vi "Protocol.Main.vi"(10 "Parameters":variant, 11 "Process":refnum<class "Process.lvclass">) -> ()   [LabVIEW 2015, in "J1939 Addon Engine.lvlib"]
uses:
  J1939 Addon Engine.lvlib
  <vilib>/NI/NIVS Inline Async API/_VS Inline Async API/Process/Process.lvclass
  Types/Protocol.App Settings.ctl
  Shared/Types/XNET Settings.ctl
  Shared/Types/Monitor Settings.ctl
  Types/Protocol.XNET Refs.ctl
  <vilib>/NI Veristand/Custom Device API/Block Data Reference.ctl
  <vilib>/NI Veristand/Custom Device API/Data Reference.ctl
  Types/Main.Outgoing.Frame.Settings.ctl
  Shared/Types/Outgoing Event Trigger Types.ctl
  Types/Engine.DTC Settings.ctl
  Shared/Types/Compiled Simulated Settings.ctl
  Types/Engine.DTC FIFOs.ctl
  <vilib>/NI/NIVS Addon Network Comm/Engine/VeriStand Comm.lvclass/VeriStand Comm.ctl
  <vilib>/NI/NIVS Inline Async API/_VS Inline Async API/Process/Process.lvclass/Process.ctl
  Protocol.Read Queued Processed Outgoing Messages.vi
  Protocol.Convert Frame to NI-XNET CAN Frame.vi
  <vilib>/NI/NIVS Inline Async API/_VS Inline Async API/Process/Methods/Async.Processes.Report.vi
  Protocol.Process Incoming Messages.vi
  <vilib>/NI/NIVS Addon Network Comm/Engine/_SubVIs/Comm Connection Engine.vi
  <vilib>/NI/NIVS Addon Network Comm/Engine/_SubVIs/Comm Command Engine.vi
  Protocol.Process J1939 Incoming Messages.vi
  Protocol.RQST Lookup Table Act.vi
  <vilib>/NI/NIVS Addon Network Comm/Engine/Comm API/Read Command.vi
  Protocol.RQST Wait on Response.vi
  Protocol.RQST Wait on Multiple Requests.vi
  Shared/J1939 Utilities/Common Conversions.vi
  Shared/J1939 Utilities/SubVIs/Convert CAN Arb ID to J1939 ID.vi
  Protocol.Address Lookup Table Action.vi
  <vilib>/NI/NIVS Addon Network Comm/Engine/Comm API/Respond to Command.vi
  <vilib>/NI/NIVS Inline Async API/_VS Inline Async API/Error Handling Process/SubVIs/Error.ConvertArray.vi
  Protocol.Filter by Device Address.vi
  Protocol.Process Incoming Messages by PDU F.vi
  <vilib>/NI/STM/Connection Manager/TCP/Advanced/TCP Connection Manager (By Reference).vi
  <vilib>/Utility/error.llb/Clear Errors.vi
  <vilib>/NI/STM/Get Connection Reference.vi
  <vilib>/NI/STM/TCP/Get Connection Reference (TCP).vi
  <vilib>/NI/STM/Read Meta Data.vi
  <vilib>/NI/STM/TCP/Read Meta Data (TCP Ref).vi
  <vilib>/NI/AMC/Send Local Message.vi
  <vilib>/NI/Tools/Keyed Array/Add.vi
  <vilib>/NI/AMC/Read Next Message.vi
  <vilib>/NI/STM/Connection Manager/TCP/Advanced/TCP Check Connection (By Reference).vi
  Protocol.J1939 Filter by Device Address.vi
  <vilib>/NI/Tools/Keyed Array/Index.vi
  Shared/J1939 Utilities/Common Messages.vi
  Shared/J1939 Utilities/SubVIs/Request.vi
  Protocol.Parse Message Type.vi
  Protocol.RQST Look for Response.vi
  Shared/J1939 Utilities/SubVIs/Convert J1939 ID to CAN Arb ID.vi
  Shared/J1939 Utilities/SubVIs/Convert CAN Data (U32) to U8.vi
  Protocol.Get Simulated Previously Active DTCs.vi
  Protocol.Get Simulated Active DTCs.vi
  Shared/J1939 Utilities/SubVIs/Acknowledgement.vi
  Protocol.Send Reset Previously Active DTC to Main.vi
  Protocol.Send Reset Active DTC to Main.vi
  Protocol.Convert Signals to Frame by ID.vi
  <vilib>/NI/STM/SubVIs/Generate STM Error.vi
  <vilib>/NI/AMC/Create Single Message.vi
  <vilib>/NI/AMC/Update Message Routing Info.vi
  <vilib>/NI/Tools/Keyed Array/Map String.vi
  <vilib>/NI/AMC/Read Termination Message.vi
  Protocol.Convert Data to DTC Frame.vi
  <vilib>/NI/Tools/String/Get Case Matching.vi
  <vilib>/NI Veristand/Custom Device Tools/Custom Device Utility Library/NI VeriStand - Print Debug String.vi
  <vilib>/xnet/xnet.llb/XNET Clear.vi
  <vilib>/NI/NIVS Addon Network Comm/Engine/Process/Close Comm Refs.vi
  Protocol.Close References.vi
  <vilib>/xnet/xnet.llb/XNET Write.vi
  <vilib>/xnet/xnet.llb/XNET Write (Frame CAN).vi
  Protocol.Address Lookup Table.vi
  <vilib>/xnet/xnet.llb/XNET Convert.vi
  <vilib>/xnet/xnet.llb/XNET Convert (Signal to Frame CAN).vi
  <vilib>/xnet/xnet.llb/XNET Create Session.vi
  <vilib>/xnet/xnet.llb/XNET Create Session (Conversion).vi
  Protocol.RQST Lookup Table.vi
  <vilib>/xnet/xnet.llb/XNET Read.vi
  <vilib>/xnet/xnet.llb/XNET Read (Frame CAN).vi
  <vilib>/NI/STM/TCP/Read Meta Data (TCP Clst).vi
  <vilib>/NI/AMC/Destroy Message Queue.vi
  <vilib>/NI/STM/Write Message.vi
  <vilib>/NI/STM/TCP/Write Message (TCP).vi
  <vilib>/NI/AMC/Globals.vi
  <vilib>/NI/AMC/Send Message.vi
  <vilib>/NI/AMC/Create Message Queue.vi
  <vilib>/NI/NIVS Addon Network Comm/Shared/Comm Constants.vi
  <vilib>/NI/STM/Read Message.vi
  <vilib>/NI/STM/TCP/Read Message (TCP).vi
  <vilib>/xnet/xnet.llb/XNET Read (State CAN Comm).vi
  <vilib>/Utility/error.llb/Error Cluster From Error Code.vi
  <vilib>/NI/NIVS Addon Network Comm/Engine/VeriStand Comm.lvclass
  Shared/J1939 Addon Shared.lvlib
  <vilib>/NI VeriStand/Custom Device API/Custom Device API.lvlib
panel:
  out "error out":errorcluster
  # "CONTROL & MONITORING"
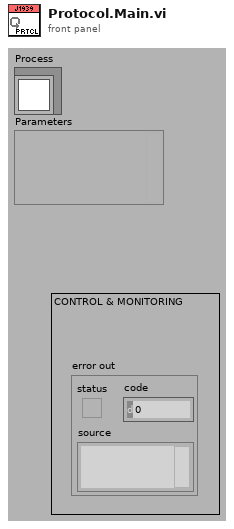
[diagram p1: front panel]
types:
  T1 = typedef "J1939 Addon Engine.lvlib/Protocol.App Settings.ctl" = cluster{"Name":string, "XNET.Settings":T2, "Monitor.Network":T3, "Data":T4[], "DTCs":T9[], "Sim.Nodes.LUT":variant, "Data.LUT":variant}
  T2 = typedef "J1939 Addon Shared.lvlib/XNET Settings.ctl" = cluster{"Database":refnum<k21>, "Cluster":refnum<k21>, "Port":string, "Baud rate [Bd]":u32, "Termination":u32, "Incoming Decimation":u32, "Outgoing Decimation":u32}
  T3 = typedef "J1939 Addon Shared.lvlib/Monitor Settings.ctl" = cluster{"Address":u8, "Name":u64, "Include DA":bool}
  T4 = typedef "J1939 Addon Engine.lvlib/Protocol.XNET Refs.ctl" = cluster{"Network":T3, "Incoming.Use":bool, "Incoming.Session":refnum<k21>, "Incoming.Refs":T5[], "Incoming.Values":dbl[], "Outgoing.Frames":T7[], "Outgoing.Initialize":bool, "Outgoing.Refs":T5[], "Outgoing.Values":dbl[], "Request.Table":refnum<k33>, "Timing.Use":bool, "Timing.Index":i32[], "Timing.Refs":T5[], "Timing.Values":dbl[], "Disable.Refs":T5[], "Disable.Values":dbl[], "Trigger.Refs":T5[], "Trigger.Values":dbl[]}
  T5 = typedef "Custom Device API.lvlib/Block Data Reference.ctl" = cluster{"Data Reference":T6, "Offset":u64, "Length":u64}
  T6 = typedef "Custom Device API.lvlib/Data Reference.ctl" = i32
  T7 = typedef "J1939 Addon Engine.lvlib/Main.Outgoing.Frame.Settings.ctl" = cluster{"Offset":u32, "Length":u32, "Cyclic":bool, "Disable.Index":i32, "Disable":bool, "Trigger":T8, "Trigger.Index":i32, "Session":refnum<k21>}
  T8 = typedef "J1939 Addon Shared.lvlib/Outgoing Event Trigger Types.ctl" = enum16{"Channel value change", "Trigger channel (not zero)", "Channel value change or trigger channel (not zero)", "Trigger channel (any value change)", "Channel value change or trigger channel (any value change)"}
  T9 = typedef "J1939 Addon Engine.lvlib/Engine.DTC Settings.ctl" = cluster{"Data":T10, "FIFOs":T11}
  T10 = typedef "J1939 Addon Shared.lvlib/Compiled Simulated Settings.ctl" = cluster{"DM1.Ref":T5[], "DM1.Value":dbl[], "DM1.Enable.Ref":T5[], "DM1.Enable.Value":dbl[], "DM2.Ref":T5[], "DM2.Value":dbl[], "DM2.Enable.Ref":T5[], "DM2.Enable.Value":dbl[]}
  T11 = typedef "J1939 Addon Engine.lvlib/Engine.DTC FIFOs.ctl" = cluster{"DM1.Data":refnum<k33>, "DM1.Enable":refnum<k33>, "DM2.Data":refnum<k33>, "DM2.Enable":refnum<k33>, "DM1.Reset":refnum<k33>, "DM2.Reset":refnum<k33>}
  T12 = typedef "J1939 Addon Engine.lvlib/Protocol.Configuration.ctl" = cluster{"Refs":T13, "XNET":T16, "Comm":refnum<class "VeriStand Comm.lvclass">, "Process":refnum<class "Process.lvclass">, "Name":string, "InternalCmd":T17, "InternalResp":T18, "Resp.Data":dbl[]}
  T13 = typedef "J1939 Addon Engine.lvlib/Protocol.Refs.ctl" = cluster{"Processed Outgoing":refnum<queue>, "Simulated Addresses LUT":variant, "Data LUT":variant, "RequestDataTables":refnum<k33>[], "RQST":T14, "Address LUT":T15, "Addresses":u8[], "Monitor Address":u8}
  T14 = typedef "J1939 Addon Engine.lvlib/Protocol.RQST Lookup Table Reference.ctl" = refnum<data-value>
  T15 = typedef "J1939 Addon Engine.lvlib/Protocol.Address Table Reference.ctl" = refnum<data-value>
  T16 = typedef "J1939 Addon Engine.lvlib/Protocol.XNET Settings.ctl" = cluster{"Raw CAN In":refnum<k21>, "Raw Frames out":refnum<k21>[], "Raw J1939 In":refnum<k21>}
  T17 = typedef "Data Access Engine.lvlib/Data Access Engine.lvclass/Read.DVR.ctl" = refnum<data-value>
  T18 = typedef "Data Access Engine.lvlib/Data Access Engine.lvclass/Write.DVR.ctl" = refnum<data-value>
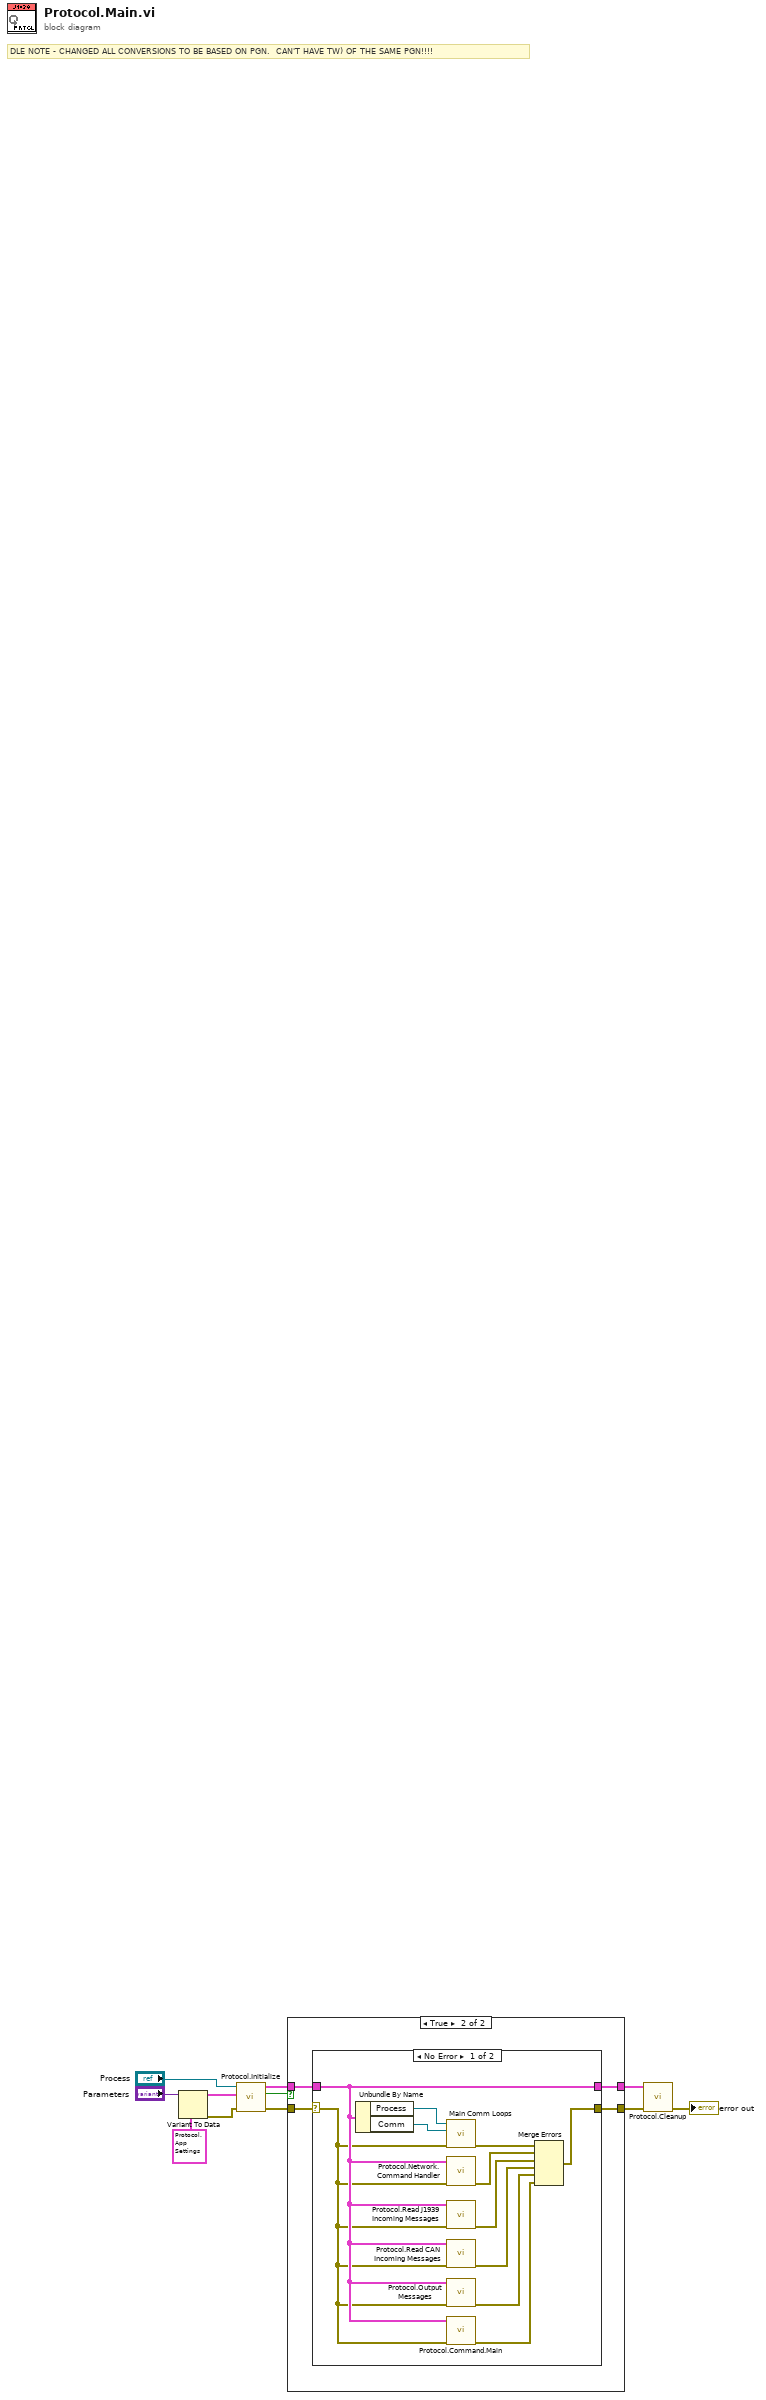
[diagram p0: block diagram]
diagram:
  # "DLE NOTE - CHANGED ALL CONVERSIONS TO BE BASED ON PGN.  CAN'T HAVE TW) OF THE SAME PGN!!!!"
  n1 = Variant To Data(type=T1 {"Name"="", "XNET.Settings"={"Database"="", "Cluster"="", "Port"="", "Baud rate [Bd]"=0, "Termination"=0, "Incoming Decimation"=0, "Outgoing Decimation"=1}, "Monitor.Network"={"Address"=0, "Name"=0, "Include DA"=FALSE}, "Data"=[], "DTCs"=[], "Sim.Nodes.LUT"=variant, "Data.LUT"=variant} ("Parameters"), Variant="Parameters") -> (data=w1:T1, error out=w2:errorcluster)  [unwired: 1 in]
  n2 = call "Protocol.Initialize.vi"("error in (no error)"=w2, "Parameters in"=w1, "Process"="Process") -> ("error out"=w11:errorcluster, "Notification"=w8:bool, "J1939 Main Configuration"=w7:T12)  [unwired: 6 in]
  n3 = case shown="True" w8 {
    tunnel: w11 -> [w13 w14]
    tunnel: [w13 w17] -> w10
    tunnel: w7 -> [w12 w15]
    tunnel: [w12 w16] -> w6
    frame False {
    }
    frame True {
      n4 = case shown="No Error" w14 {
        selector: w14 -> [w19 w30]
        tunnel: [w28 w30] -> w17
        tunnel: w15 -> [w20 w29]
        tunnel: [w20 w29] -> w16
        frame No Error {
          n5 = Unbundle By Name(w20) -> ("Process"=w24:refnum<class "Process.lvclass">, "Comm"=w25:refnum<class "VeriStand Comm.lvclass">)
          n6 = call <vilib>:"Main Comm Loops.vi"("error in (no error)"=w19, "Comm.lvclass"=w25, "Process"=w24) -> ("error out"=w22:errorcluster)  [unwired: 8 in]
          n7 = call "Protocol.Network.Command Handler.vi"("error in (no error)"=w19, "J1939 Main Configuration"=w20) -> ("error out"=w23:errorcluster)  [unwired: 9 in]
          n8 = call "Protocol.Read J1939 Incoming Messages.vi"("error in (no error)"=w19, "J1939 Main Configuration"=w20) -> ("error out"=w21:errorcluster)  [unwired: 9 in]
          n9 = call "Protocol.Read CAN Incoming Messages.vi"("error in (no error)"=w19, "J1939 Main Configuration"=w20) -> ("error out"=w27:errorcluster)  [unwired: 9 in]
          n10 = call "Protocol.Output Messages.vi"("error in (no error)"=w19, "J1939 Main Configuration"=w20) -> ("error out"=w26:errorcluster)  [unwired: 9 in]
          n11 = call "Protocol.Command.Main.vi"("Error"=w19, "J1939 Main Configuration"=w20) -> ("error out"=w18:errorcluster)  [unwired: 9 in]
          n12 = Merge Errors(w22, w23, w21, w27, w26, w18) -> (w28:errorcluster)
        }
        frame Error {
        }
      }
    }
  }
  n13 = call "Protocol.Cleanup.vi"("error in (no error)"=w10, "J1939 Main Configuration"=w6) -> ("error out"=→"error out":errorcluster)  [unwired: 9 in]
